vi "ReadDIs.vi"(8 "error in (no error)":errorcluster, 10 "Digital Inputs":T1, 11 "VISA resource name":refnum<visa-resource-name>) -> (0 "error out":errorcluster, 2 "DIStatus":bool, 3 "VISA resource name out":refnum<visa-resource-name>)   [LabVIEW 2022 SP3, in "HandsOnPi2040.lvlib"]
uses:
  <instrlib>/HandsOnPi2040/HandsOnPi2040.lvlib
  <instrlib>/HandsOnPi2040/Public/DigIns.ctl
  <instrlib>/HandsOnPi2040/cti-drivers-lv-visa-main/CTI-Visa/CTI-Visa.lvlib
panel:
  # "Output"
  # "Input"
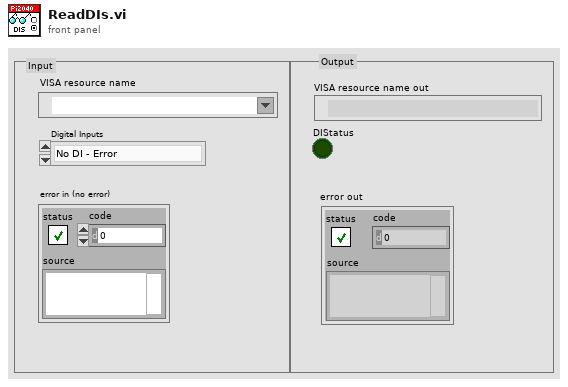
[diagram p1: front panel]
types:
  T1 = typedef "HandsOnPi2040.lvlib/DigIns.ctl" = enum16{"No DI - Error", "DI1", "DI2", "DI3", "DI4"}
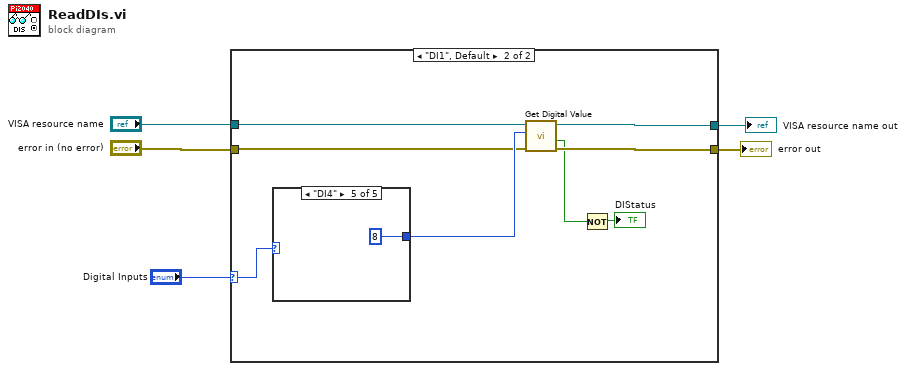
[diagram p0: block diagram]
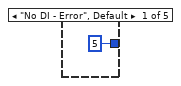
[diagram p3: hidden frame]
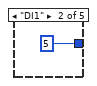
[diagram p4: hidden frame]
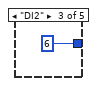
[diagram p5: hidden frame]
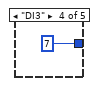
[diagram p6: hidden frame]
diagram:
  n1 = case shown="\"DI1\", Default" "Digital Inputs" {
    selector: "Digital Inputs" -> [_ w12]
    tunnel: "VISA resource name" -> [w6 w10]
    tunnel: "error in (no error)" -> [w7 w9]
    tunnel: [w6 w14] -> w5
    tunnel: [w7 w15] -> w4
    frame "No DI - Error" {
    }
    frame "DI1", Default {
      n2 = case shown="\"DI4\"" w12 {
        tunnel: [5 ("Channel") 5 ("Channel") 6 ("Channel") 7 ("Channel") 8 ("Channel")] -> w11
        frame "No DI - Error", Default {
        }
        frame "DI1" {
        }
        frame "DI2" {
        }
        frame "DI3" {
        }
        frame "DI4" {
        }
      }
      n3 = call <instrlib>:"Get Digital Value.vi"("error in (no error)"=w9, "Channel"=w11, "VISA resource name in"=w10) -> ("error out"=w15:errorcluster, "Value"=w13:bool, "VISA resource name"=w14:refnum<visa-resource-name>)  [unwired: 6 in]
      n4 = Not(x=w13) -> (.not. x?=→"DIStatus":bool)
    }
  }
  "VISA resource name out" <- w5
  "error out" <- w4
